vi "FTW-Logger-Destroy.vi"(0 "FTW Logger":refnum<class "FTW-Logger-Core.lvclass">, 11 "error in":errorcluster) -> (15 "error out":errorcluster)   [LabVIEW 2012, in "FTW-Actor.lvlib" / "FTW-Logger-Core.lvclass"]
uses:
  FTW-Logger-Core.lvclass
panel:
  # "Inputs"
  # "Outputs"
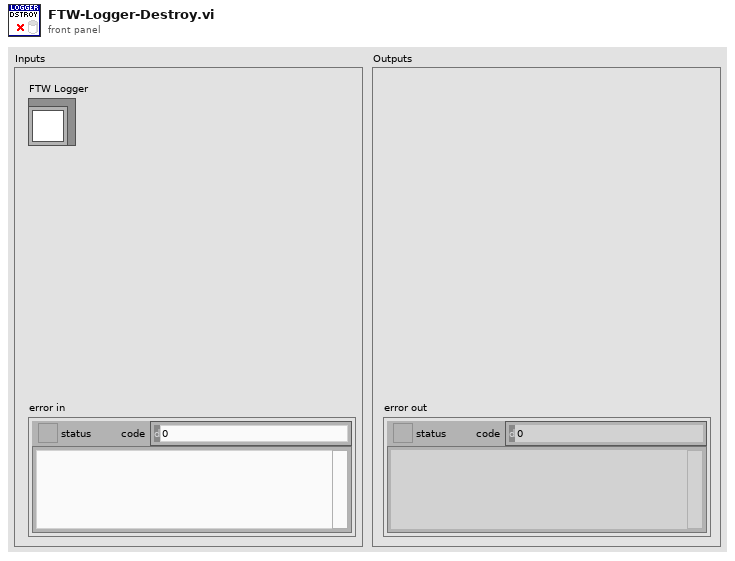
[diagram p1: front panel]
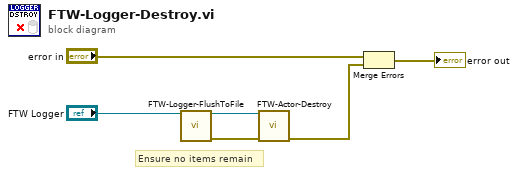
[diagram p0: block diagram]
diagram:
  # "Ensure no items remain"
  n1 = call "FTW-Logger-FlushToFile.vi"("Event Logger"="FTW Logger") -> ("Event Logger out"=w3:refnum<class "FTW-Logger-Core.lvclass">, "error out"=w2:errorcluster)  [unwired: 13 in]
  n2 = call-dynamic "FTW-Actor-Destroy.vi"("FTW Actor Instance"=w3, "error in"=w2) -> ("error out"=w1:errorcluster)  [unwired: 13 in]
  n3 = Merge Errors("error in", w1) -> (→"error out":errorcluster)
